vi "test Loopback_Complex.vi"(8 "error in":errorcluster, 11 "TestCase in":refnum<class "Single Core Complex Loopback.lvclass">) -> (0 "error out":errorcluster, 3 "TestCase out":refnum<class "Single Core Complex Loopback.lvclass">)   [LabVIEW 2020, in "Single Core Complex Loopback.lvclass"]
uses:
  Single Core Complex Loopback.lvclass
  C:/Git/niveristand-custom-device-testing-tools/VeriStandTestCase/VeriStandTestCase.lvclass
  <vilib>/numeric/Random Number (Range) DBL.vi
  <vilib>/NI VeriStand/Execution/Workspace/NI VeriStand - Get Single Channel Value.vi
  <vilib>/addons/_JKI Toolkits/VI Tester/TestCase.llb/TestCase.lvclass
  niveristand-custom-device-testing-tools/VeriStandTestUtilities/VeriStandTestUtilities.lvlib
  <vilib>/NI VeriStand/Execution/Workspace/NI_VS Workspace ExecutionAPI.lvlib
  C:/Program Files (x86)/National Instruments/LabVIEW 2020/vi.lib/addons/_JKI Toolkits/VI Tester/TestCase.llb/TestCase.lvclass
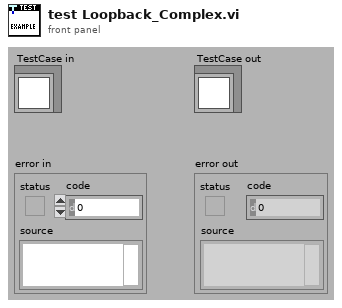
[diagram p1: front panel]
types:
  T1 = typedef "NI_VS Workspace ExecutionAPI.lvlib/WorkspaceAPI.ctl" = refnum<k24>
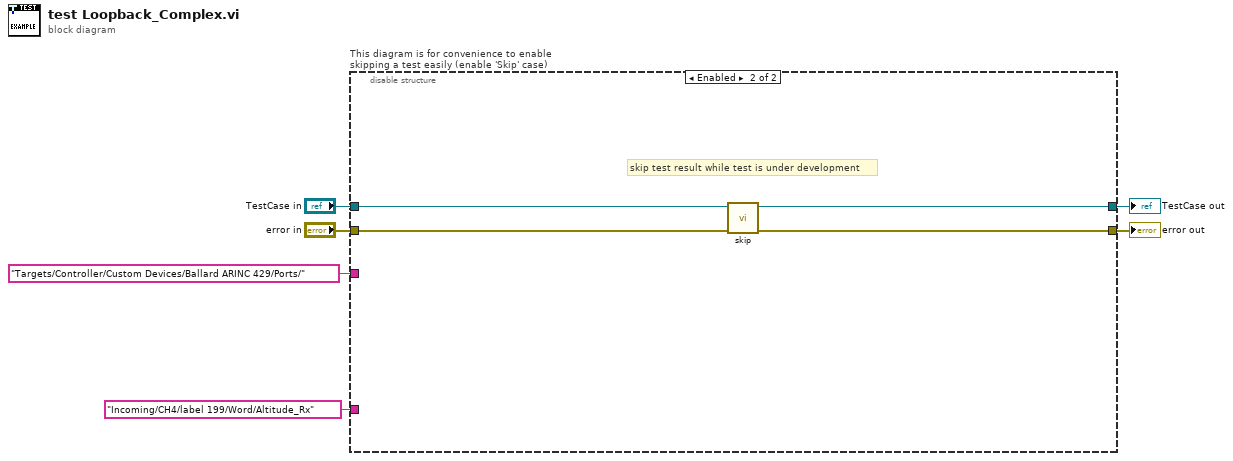
[diagram p0: block diagram]
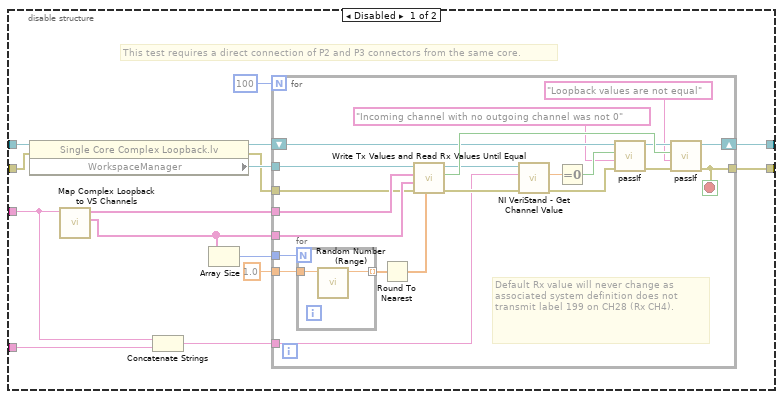
[diagram p2: hidden frame]
diagram:
  n1 = disable-structure "This diagram is for convenience to enable skipping a test easily (enable 'Skip' case)" shown="Enabled" {
    disable-tunnel: "TestCase in" -> [w14 w49]
    disable-tunnel: [w8 w47] -> w3
    disable-tunnel: [w7 w48] -> w5
    disable-tunnel: "error in" -> [w9 w46]
    disable-tunnel: "Targets/Controller/Custom Devices/Ballard ARINC 429/Ports/" ("Channel") -> [w11 _]
    disable-tunnel: "Incoming/CH4/label 199/Word/Altitude_Rx" ("Channel") -> [w10 _]
    frame Disabled {
      # "This test requires a direct connection of P2 and P3 connectors from the same core."
      n2 = property class="Single Core Complex Loopback.lv"(reference=w14, error in=w9) -> (reference out=w19:refnum<class "Single Core Complex Loopback.lvclass">, error out=w20:errorcluster, "WorkspaceManager"=w21:T1)
      n3 = call "Map Complex Loopback to VS Channels.vi"("Base Path to Ports"=w11) -> ("Rx Channel Array"=w13:string[], "Tx Channel Array"=w12:string[])  [unwired: 9 in]
      n4 = Concatenate Strings(w11, w10) -> (w16:string)
      n5 = Array Size(array=w13) -> (size(s)=w15:i32)
      n6 = for {
        N: 100 ("x") -> [_]
        tunnel: w12 -> [w38]
        tunnel: w21 -> [w39]
        tunnel: w20 -> [w35]
        tunnel: w13 -> [w37]
        shift-right: [w43] -> w8
        shift-left: w19 -> [w27]
        tunnel: [w42] -> w7
        tunnel: 1.0 ("upper bound (100)") -> [w40]
        tunnel: w16 -> [w31]
        tunnel: w15 -> [w24]
        stop <- w42 stop-if-true
        # "Default Rx value will never change as associated system definition does not transmit label 199 on CH28 (Rx CH4)."
        n7 = for {
          N: w24 -> [_]
          tunnel: [w45] -> w41 mode=indexing
          tunnel: w40 -> [w44]
          n8 = call-poly <vilib>:"Random Number (Range).vi"("upper bound (100)"=w44) -> ("number"=w45:dbl)  [unwired: 10 in]
        }
        n9 = Round To Nearest(number=w41) -> (nearest integer value=w34:dbl[])
        n10 = call "Write Tx Values and Read Rx Values Until Equal.vi"("Tx values"=w34, "error in"=w35, "Rx aliases"=w37, "Tx aliases"=w38, "workspace manager in"=w39) -> ("error out"=w32:errorcluster, "values equal"=w36:bool, "workspace manager out"=w33:T1)  [unwired: 4 in]
        n11 = call-poly <vilib>:"NI VeriStand - Get Channel Value.vi"("error in (no error)"=w32, "Channel"=w31, "WorkspaceManager in"=w33) -> ("error out"=w29:errorcluster, "Value"=w30:dbl)  [unwired: 6 in, 1 out]
        n12 = Equal To 0?(x=w30) -> (x = 0?=w25:bool)
        n13 = call-dynamic "passIf.vi"("error in (no error)"=w29, "message (\"\")"="Incoming channel with no outgoing channel was not 0" ("message (\"\")"), "pass"=w25, "TestCase in"=w27) -> ("error out"=w28:errorcluster, "TestCase out"=w26:refnum<class "Single Core Complex Loopback.lvclass">)  [unwired: 6 in]
        n14 = call-dynamic "passIf.vi"("error in (no error)"=w28, "message (\"\")"="Loopback values are not equal" ("message (\"\")"), "pass"=w36, "TestCase in"=w26) -> ("error out"=w42:errorcluster, "TestCase out"=w43:refnum<class "Single Core Complex Loopback.lvclass">)  [unwired: 6 in]
      }
    }
    frame Enabled {
      # "skip test result while test is under development"
      n15 = call <vilib>:"skip.vi"("error in (no error)"=w46, "TestCase in"=w49) -> ("error out"=w48:errorcluster, "TestCase out"=w47:refnum<class "Single Core Complex Loopback.lvclass">)  [unwired: 8 in]
    }
  }
  "error out" <- w5
  "TestCase out" <- w3
